vi "DN4_CheckChannelCount.vi"(3 "error out":errorcluster, 5 "channel count":i32) -> (0 "error IO":errorcluster, 2 "greater than 1?":bool)   [LabVIEW 2020]
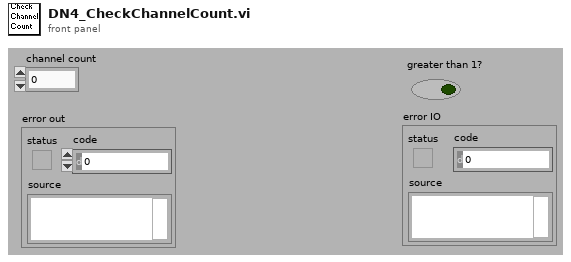
[diagram p1: front panel]
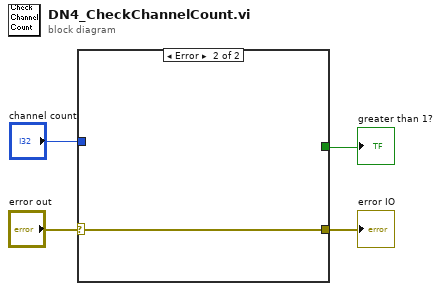
[diagram p0: block diagram]
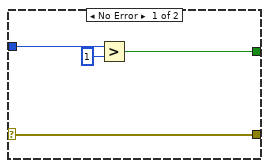
[diagram p2: hidden frame]
diagram:
  n1 = case shown="Error" "error out" {
    selector: "error out" -> [w5 w9]
    tunnel: "channel count" -> [w7 _]
    tunnel: [w6 _] -> w2
    tunnel: [w5 w9] -> w1
    frame No Error {
      n2 = Greater?(x=w7, y=1) -> (0:w6:bool)
    }
    frame Error {
    }
  }
  "greater than 1?" <- w2
  "error IO" <- w1
